vi "Read Device.vi"(8 "error in (no error)":errorcluster, 11 "DAC in":refnum<class "DAC.lvclass">) -> (0 "error out":errorcluster, 2 "Device":string caption="DAC Device", 3 "DAC out":refnum<class "DAC.lvclass">)   [LabVIEW 2019, in "DAC.lvlib" / "DAC.lvclass"]
uses:
  DAC.lvclass
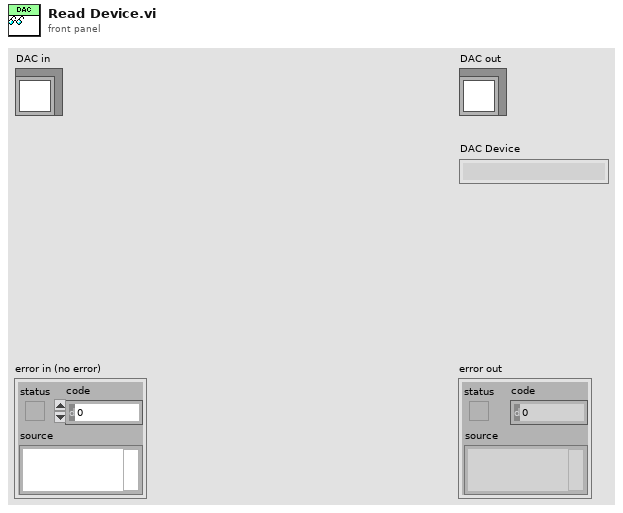
[diagram p1: front panel]
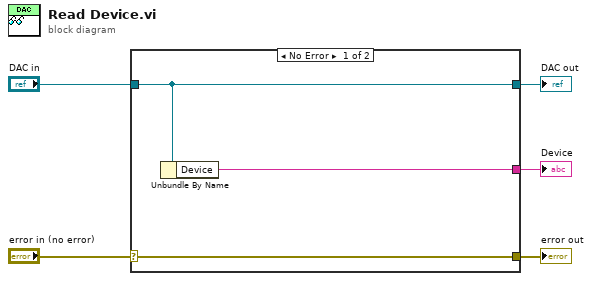
[diagram p0: block diagram]
diagram:
  n1 = case shown="No Error" "error in (no error)" {
    selector: "error in (no error)" -> [w8 w9]
    tunnel: [w8 w9] -> w4
    tunnel: [w7 w10] -> w2
    tunnel: "DAC in" -> [w7 w10]
    tunnel: [w6 _] -> w1
    frame No Error {
      n2 = Unbundle By Name(w7) -> ("Device"=w6:string)
    }
    frame Error {
    }
  }
  "error out" <- w4
  "DAC out" <- w2
  "Device" <- w1
